vi "remove.vi"() -> ()   [LabVIEW 2018]
panel:
  in  "stop":bool
  out "Array":u16[](array[numeric])
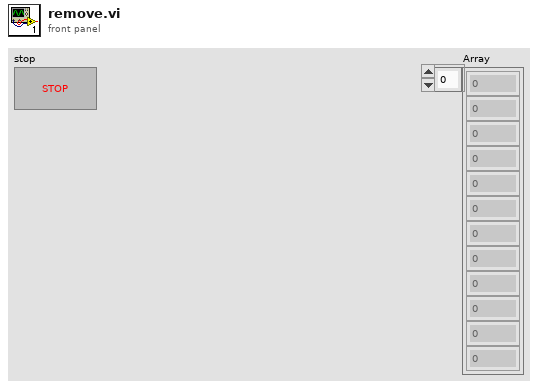
[diagram p1: front panel]
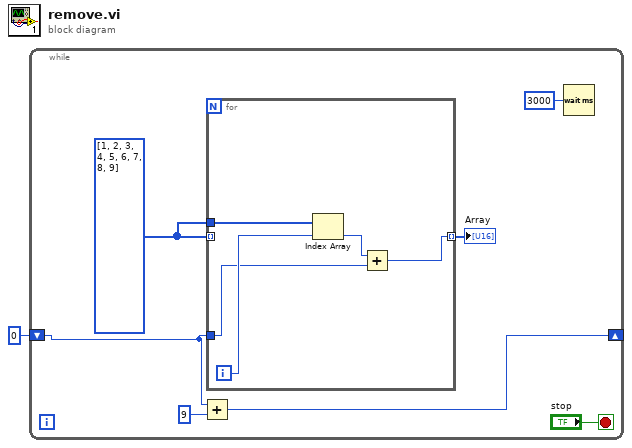
[diagram p0: block diagram]
diagram:
  n1 = while {
    shift-right: [w2] -> _
    shift-left: 0 -> [w4]
    stop <- "stop" stop-if-true
    w5 = u16[] [1, 2, 3, 4, 5, 6, 7, 8, 9]
    n2 = Add(x=w4, y=9) -> (x+y=w2:i32)
    n3 = for {
      tunnel: w5 -> [_] mode=indexing
      tunnel: [w9] -> w8 mode=indexing
      tunnel: w4 -> [w10]
      tunnel: w5 -> [w13]
      i -> [w12]
      n4 = Index Array(array=w13, index=w12) -> (element=w11:u16)
      n5 = Add(x=w11, y=w10) -> (x+y=w9:i32)
    }
    "Array" <- w8
    n6 = Wait (ms)(milliseconds to wait=u32 3000) -> ()  [unwired: 1 out]
  }
